vi "Create Sysdef Tree from DB Channel Clusters.vi"(7 "Autocreate Rx timestamp chans?":bool, 8 "error in":errorcluster, 10 "Channels to create":T2 {"speed" items=["OWL429_HIGH_SPEED_CHANNEL", "OWL429_LOW_SPEED_CHANNEL"]; "Labels"."scheduleBuildUnit" items=["Millisecond", "Microsecond"]}, 11 "Device Ptr":u64) -> (0 "error out":errorcluster, 3 "Device Ptr dup":u64)   [LabVIEW 2017, in "Ballard Arinc-429 System Explorer.lvlib"]
uses:
  Ballard Arinc-429 System Explorer.lvlib
  Controls/Ballard_Channel Array.ctl
  Controls/Ballard_Channel.ctl
  Controls/Ballard_Label.ctl
  Controls/Ballard_Word.ctl
  Controls/ARINCParam.ctl
  Shared/Controls and Global/TransferType.ctl
  Controls/Channel_direction.ctl
  Controls/Channel Speed.ctl
  Build Label Properties.vi
  <vilib>/NI Veristand/Custom Device API/NI VeriStand - Add Custom Device Channel.vi
  <vilib>/NI Veristand/Custom Device API/NI VeriStand - Set Item Description.vi
  Create Tx Word Description.vi
  Shared/Controls and Global/Global.vi
  <vilib>/NI Veristand/Custom Device Tools/Custom Device Utility Library/NI VeriStand - Search for Item by GUID.vi
  <vilib>/NI Veristand/Custom Device API/Custom Device API.lvlib
  Shared/Ballard Arinc-429 Shared.lvlib
  <vilib>/NI Veristand/Custom Device Tools/Custom Device Utility Library/Custom Device Utility Library.lvlib
panel:
  out "direction":T1
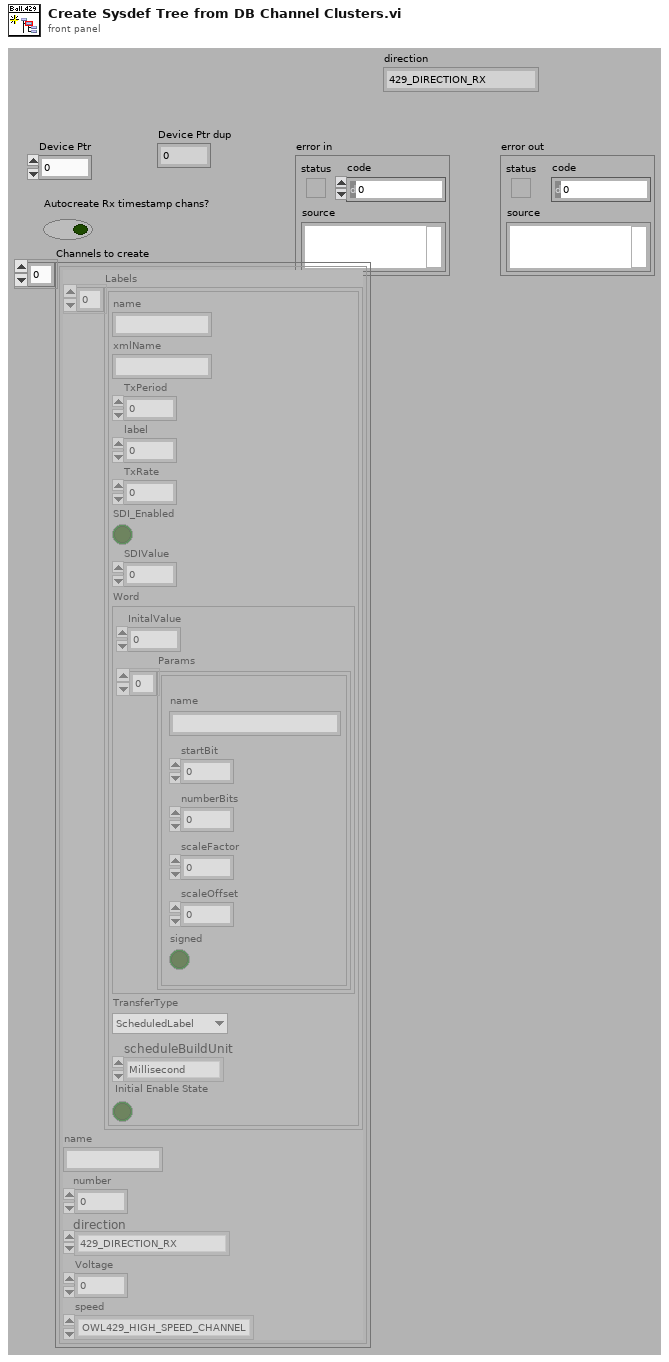
[diagram p1: front panel]
types:
  T1 = typedef "Ballard Arinc-429 System Explorer.lvlib/Channel_direction.ctl" = enum16{"429_DIRECTION_RX", "429_DIRECTION_TX"}
  T2 = typedef "Ballard Arinc-429 System Explorer.lvlib/Ballard_Channel Array.ctl" = T3[]
  T3 = typedef "Ballard Arinc-429 System Explorer.lvlib/Ballard_Channel.ctl" = cluster{"Labels":T4[], "name":string, "number":u8, "direction":T1, "Voltage":dbl, "speed":T8}
  T4 = typedef "Ballard Arinc-429 System Explorer.lvlib/Ballard_Label.ctl" = cluster{"name":string, "xmlName":string, "TxPeriod":u32, "label":u32, "TxRate":dbl, "SDI_Enabled":bool, "SDIValue":u8, "Word":T5, "TransferType":T7, "scheduleBuildUnit":i32, "Initial Enable State":bool}
  T5 = typedef "Ballard Arinc-429 System Explorer.lvlib/Ballard_Word.ctl" = cluster{"InitalValue":u32, "Params":T6[]}
  T6 = typedef "Ballard Arinc-429 System Explorer.lvlib/ARINCParam.ctl" = cluster{"name":string, "startBit":i32, "numberBits":i32, "scaleFactor":dbl, "scaleOffset":dbl, "signed":bool}
  T7 = typedef "Ballard Arinc-429 Shared.lvlib/TransferType.ctl" = enum16{"ScheduledLabel", "Acyclic", "Block", "Strobe"}
  T8 = typedef "Ballard Arinc-429 System Explorer.lvlib/Channel Speed.ctl" = i32
  T9 = typedef "Custom Device API.lvlib/Custom Device Item Ref.ctl" = u64
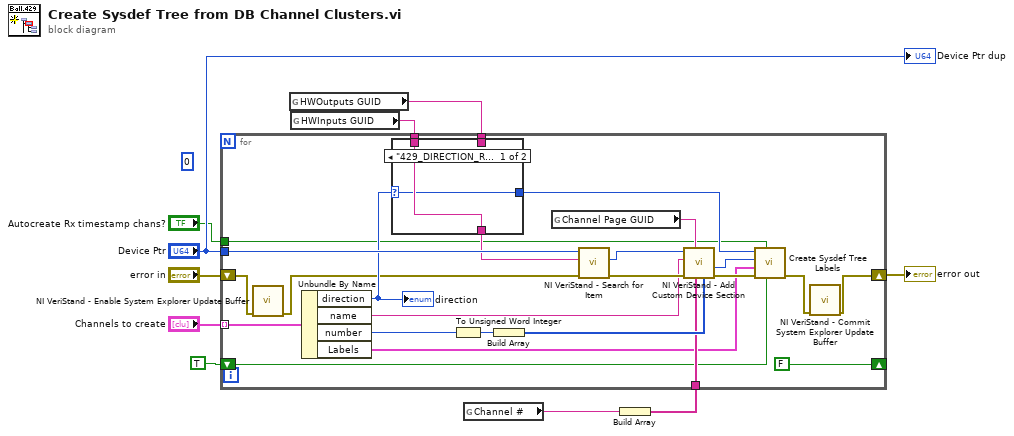
[diagram p0: block diagram]
diagram:
  (unwired) 0
  n1 = global read "Global.vi" "HWOutputs GUID"() -> (w8:string)
  n2 = global read "Global.vi" "HWInputs GUID"() -> (w9:string)
  n3 = global read "Global.vi" "Channel #"() -> (w6:string)
  n4 = Build Array(w6) -> (w7:string[])
  n5 = for {
    tunnel: "Device Ptr" -> [w31]
    shift-right: [w11] -> w4
    shift-left: "error in" -> [w14]
    tunnel: "Channels to create" -> [w32] mode=indexing
    tunnel: w7 -> [w26]
    tunnel: w8 -> [w21]
    tunnel: w9 -> [w22]
    shift-right: [FALSE] -> _
    shift-left: TRUE -> [w17]
    tunnel: "Autocreate Rx timestamp chans?" -> [w15]
    n6 = call <vilib>:"NI VeriStand - Enable System Explorer Update Buffer.vi"("error in (no error)"=w14) -> ("error out"=w13:errorcluster)  [unwired: 10 in]
    n7 = Unbundle By Name(w32) -> ("direction"=w24:T1, "name"=w28:string, "number"=w27:u8, "Labels"=w20:T4[])
    "direction" <- w24
    n8 = case shown="\"429_DIRECTION_RX\"" w24 {
      selector: w24 -> [w36 w38]
      tunnel: [w37 w39] -> w23
      tunnel: w22 -> [w37 _]
      tunnel: w21 -> [_ w39]
      tunnel: [w36 w38] -> w19
      frame "429_DIRECTION_RX" {
      }
      frame "429_DIRECTION_TX" {
      }
    }
    n9 = To Unsigned Word Integer(number=w27) -> (unsigned 16bit integer=w25:u16)
    n10 = Build Array(w25) -> (w34:u16[])
    n11 = global read "Global.vi" "Channel Page GUID"() -> (w33:string)
    n12 = call-poly <vilib>:"NI VeriStand - Search for Item.vi"("error in"=w13, "Item GUID"=w23, "Section Ref in"=w31) -> ("error out"=w29:errorcluster, "Item Ref"=w30:T9)  [unwired: 5 in, 2 out]
    n13 = call <vilib>:"NI VeriStand - Add Custom Device Section.vi"("Property Values"=w34, "Property names"=w26, "GUID (Default Section)"=w33, "error in (no error)"=w29, "Section Name"=w28, "Parent Ref in"=w30) -> ("error out"=w35:errorcluster, "Section Ptr"=w18:T9)  [unwired: 2 in, 2 out]
    n14 = call "Create Sysdef Tree Labels.vi"("first call"=w17, "Autocreate Rx timestamp chans?"=w15, "error in"=w35, "Labels"=w20, "Section Ptr"=w18, "direction"=w19) -> ("error out"=w12:errorcluster)  [unwired: 5 in]
    n15 = call <vilib>:"NI VeriStand - Commit System Explorer Update Buffer.vi"("error in (no error)"=w12) -> ("error out"=w11:errorcluster)  [unwired: 10 in]
  }
  "error out" <- w4
  "Device Ptr dup" <- "Device Ptr"
